vi "Read write Master.vi"(8 "error in (no error)":errorcluster, 10 "ELAN data unit in":refnum<class "ELAN PDU.lvclass">, 11 "ELAN master in":refnum<class "ELAN Master.lvclass">) -> (0 "error out":errorcluster, 1 "PDU valid?":bool, 2 "ELAN data unit out":refnum<class "ELAN PDU.lvclass">, 3 "ELAN master out":refnum<class "ELAN Master.lvclass">)   [LabVIEW 2021, in "ELAN Master.lvclass"]
doc: "This VI allows a mutex for the master API without restricting any other functions. This mutex is currently unimplemented."
uses:
  ELAN Master.lvclass
  Data Unit/ELAN PC Data Unit/ELAN PDU.lvclass
  ELAN Master.lvclass/ELAN Master.ctl
  Transmission Data Unit/ELAN/ELAN Data Unit.lvclass/ELAN Data Unit.ctl
  Data Unit/ELAN PC Data Unit/ELAN PDU.lvclass/ELAN PDU.ctl
  Data Unit/ELAN PC Data Unit/Flatten PDU.vi
  Modbus_v121c/Network Interface/Serial Interface/SSC/Serial Write.vi
  Transmission Data Unit/ELAN/Calculate CRC.vi
  Data Unit/ELAN PC Data Unit/Unflatten to PDU.vi
  Transmission Data Unit/ELAN/Check For Messages.vi
  <vilib>/Utility/error.llb/Error Cluster From Error Code.vi
  Transmission Data Unit/ELAN/ELAN Data Unit.lvclass
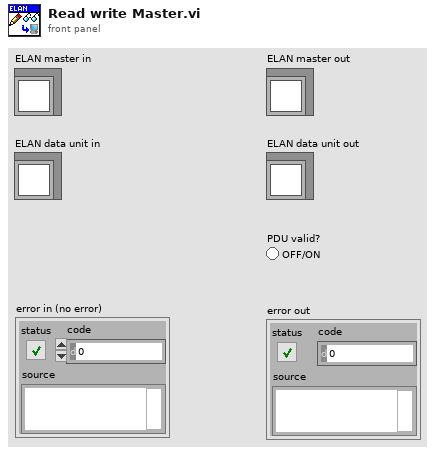
[diagram p1: front panel]
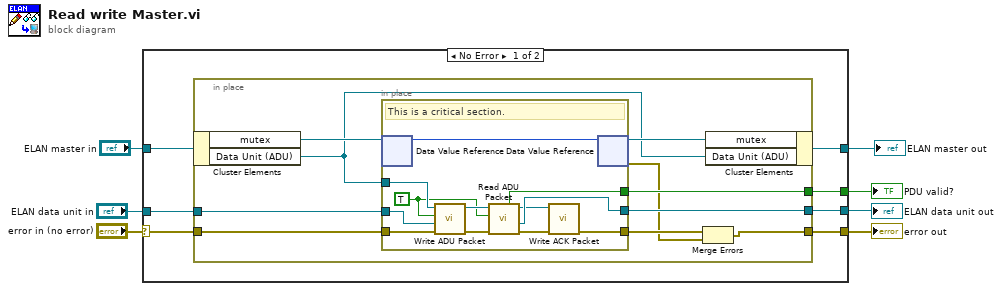
[diagram p0: block diagram]
diagram:
  n1 = case shown="No Error" "error in (no error)" {
    selector: "error in (no error)" -> [w9 w37]
    tunnel: "ELAN master in" -> [w10 w38]
    tunnel: [w8 w38] -> w6
    tunnel: "ELAN data unit in" -> [w14 w39]
    tunnel: [w13 w39] -> w4
    tunnel: [w12 w37] -> w3
    tunnel: [w11 _] -> w2
    frame No Error {
      n2 = in-place {
        in-place-border: w9 -> [w23]
        in-place-border: w14 -> [w22]
        in-place-border: [w20] -> w13
        in-place-border: [w19] -> w12
        in-place-border: [w18] -> w11
        n3 = in-place-cluster #1(w10) -> ("mutex"=w24:refnum<data-value>, "Data Unit (ADU)"=w15:refnum<class "ELAN Data Unit.lvclass">)
        n4 = in-place {
          in-place-border: w23 -> [w33]
          in-place-border: w22 -> [w32]
          in-place-border: [w26] -> w17
          in-place-border: [w28] -> w20
          in-place-border: [w31] -> w18
          in-place-border: w15 -> [w30]
          w29 = TRUE ("isMaster (f)")
          # "This is a critical section."
          n5 = in-place-dvr #2(w24) -> (w34:u8)  [unwired: 1 out]
          n6 = call "Write ADU Packet.vi"("error in"=w33, "ELAN data unit"=w32, "isMaster (f)"=w29, "ELAN data unit (ADU) in"=w30) -> ("error out"=w36:errorcluster, "ELAN data unit (ADU) out"=w35:refnum<class "ELAN Data Unit.lvclass">)  [unwired: 6 in]
          n7 = call "Read ADU Packet.vi"("error in"=w36, "isMaster (f)"=w29, "ELAN data unit (ADU) in"=w35) -> ("error out"=w27:errorcluster, "ELAN data unit (PDU)"=w28:refnum<class "ELAN PDU.lvclass">, "ELAN data unit (ADU) out"=w25:refnum<class "ELAN Data Unit.lvclass">, "PDU Valid?"=w31:bool)  [unwired: 5 in]
          n8 = call "Write ACK Packet.vi"("error in"=w27, "ELAN data unit (ADU) in"=w25) -> ("error out"=w26:errorcluster)  [unwired: 8 in, 1 out]
          n9 = in-place-dvr #2(w34) -> (w21:refnum<data-value>, w16:errorcluster)
        }
        n10 = Merge Errors(w17, w16) -> (w19:errorcluster)
        n11 = in-place-cluster #1("mutex"=w21, "Data Unit (ADU)"=w15) -> (w8:refnum<class "ELAN Master.lvclass">)
      }
    }
    frame Error {
    }
  }
  "ELAN data unit out" <- w4
  "ELAN master out" <- w6
  "error out" <- w3
  "PDU valid?" <- w2
